vi "Kamera hinten.vi"() -> (0 "Paket erkannt":bool, 1 "Barcode erkannt":bool, 2 "Paketkoordinaten":cluster{"X":dbl, "Y":dbl}, 3 "Barcode":u32)   [LabVIEW 2019]
doc: "Erkennt mit Hilfe der hiten angebrachten Kamera das Paket und den Barcode. Es gitb den Barcode aus und eine ungefähre mittige Position der Kamera."
panel:
  out "Rectangles (Shape Detection 1)":T1(array[cluster]) {"Corners"."Y" format="%.2f"; "Corners"."X" format="%.2f"}
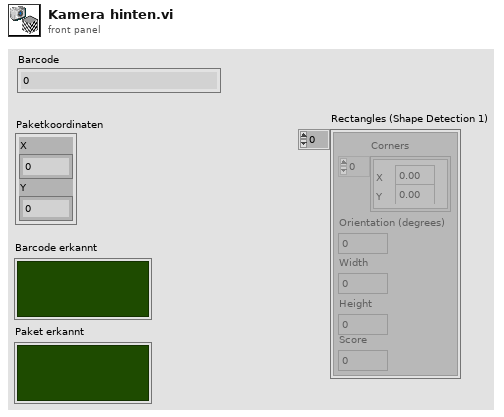
[diagram p1: front panel]
types:
  T1 = cluster{"Corners":cluster{"X":sgl, "Y":sgl}[], "Orientation (degrees)":dbl, "Width":dbl, "Height":dbl, "Score":dbl}[]
  T2 = typedef "IMAQ Image.ctl" = refnum<image>
  T3 = typedef "Edge New.ctl" = cluster{"Location (Pixel)":cluster{"X":sgl, "Y":sgl}, "Location (Real-World)":cluster{"X":sgl, "Y":sgl}, "Distance (Pixel)":dbl, "Distance (Real-World)":dbl, "Strength":dbl, "Noise":dbl, "Rising?":bool}
  T4 = cluster{"Data":string, "Special Char 1":string, "Special Char 2":string, "Checksum(s)":string, "Barcode Type":u32, "Confidence Level":sgl, "Bounding Box":cluster{"x":sgl, "y":sgl}[]}[]
  T5 = cluster{"Edge Information (Edge Detector 3)[0]":T3, "Edge Information (Edge Detector 3)[1]":T3, "Edge Information (Edge Detector 3)[2]":T3, "Edge Information (Edge Detector 3)[3]":T3, "Edge Information (Edge Detector 3)[4]":T3, "Edge Information (Edge Detector 3)[5]":T3, "Edge Information (Edge Detector 3)[6]":T3, "Edge Information (Edge Detector 3)[7]":T3, "Edge Information (Edge Detector 3)[8]":T3}
  T6 = cluster{"Barcodes (Barcode Reader 1)[0]":cluster{"Data":string, "Special Char 1":string, "Special Char 2":string, "Checksum(s)":string, "Barcode Type":u32, "Confidence Level":sgl, "Bounding Box":cluster{"x":sgl, "y":sgl}[]}, "Barcodes (Barcode Reader 1)[1]":cluster{"Data":string, "Special Char 1":string, "Special Char 2":string, "Checksum(s)":string, "Barcode Type":u32, "Confidence Level":sgl, "Bounding Box":cluster{"x":sgl, "y":sgl}[]}, "Barcodes (Barcode Reader 1)[2]":cluster{"Data":string, "Special Char 1":string, "Special Char 2":string, "Checksum(s)":string, "Barcode Type":u32, "Confidence Level":sgl, "Bounding Box":cluster{"x":sgl, "y":sgl}[]}, "Barcodes (Barcode Reader 1)[3]":cluster{"Data":string, "Special Char 1":string, "Special Char 2":string, "Checksum(s)":string, "Barcode Type":u32, "Confidence Level":sgl, "Bounding Box":cluster{"x":sgl, "y":sgl}[]}, "Barcodes (Barcode Reader 1)[4]":cluster{"Data":string, "Special Char 1":string, "Special Char 2":string, "Checksum(s)":string, "Barcode Type":u32, "Confidence Level":sgl, "Bounding Box":cluster{"x":sgl, "y":sgl}[]}, "Barcodes (Barcode Reader 1)[5]":cluster{"Data":string, "Special Char 1":string, "Special Char 2":string, "Checksum(s)":string, "Barcode Type":u32, "Confidence Level":sgl, "Bounding Box":cluster{"x":sgl, "y":sgl}[]}, "Barcodes (Barcode Reader 1)[6]":cluster{"Data":string, "Special Char 1":string, "Special Char 2":string, "Checksum(s)":string, "Barcode Type":u32, "Confidence Level":sgl, "Bounding Box":cluster{"x":sgl, "y":sgl}[]}, "Barcodes (Barcode Reader 1)[7]":cluster{"Data":string, "Special Char 1":string, "Special Char 2":string, "Checksum(s)":string, "Barcode Type":u32, "Confidence Level":sgl, "Bounding Box":cluster{"x":sgl, "y":sgl}[]}, "Barcodes (Barcode Reader 1)[8]":cluster{"Data":string, "Special Char 1":string, "Special Char 2":string, "Checksum(s)":string, "Barcode Type":u32, "Confidence Level":sgl, "Bounding Box":cluster{"x":sgl, "y":sgl}[]}}
  T7 = cluster{"Edge Information (Edge Detector 2)[0]":T3, "Edge Information (Edge Detector 2)[1]":T3, "Edge Information (Edge Detector 2)[2]":T3, "Edge Information (Edge Detector 2)[3]":T3, "Edge Information (Edge Detector 2)[4]":T3, "Edge Information (Edge Detector 2)[5]":T3, "Edge Information (Edge Detector 2)[6]":T3, "Edge Information (Edge Detector 2)[7]":T3, "Edge Information (Edge Detector 2)[8]":T3}
  T8 = cluster{"Data":string, "Special Char 1":string, "Special Char 2":string, "Checksum(s)":string, "Barcode Type":u32, "Confidence Level":sgl, "Bounding Box":cluster{"x":sgl, "y":sgl}[]}
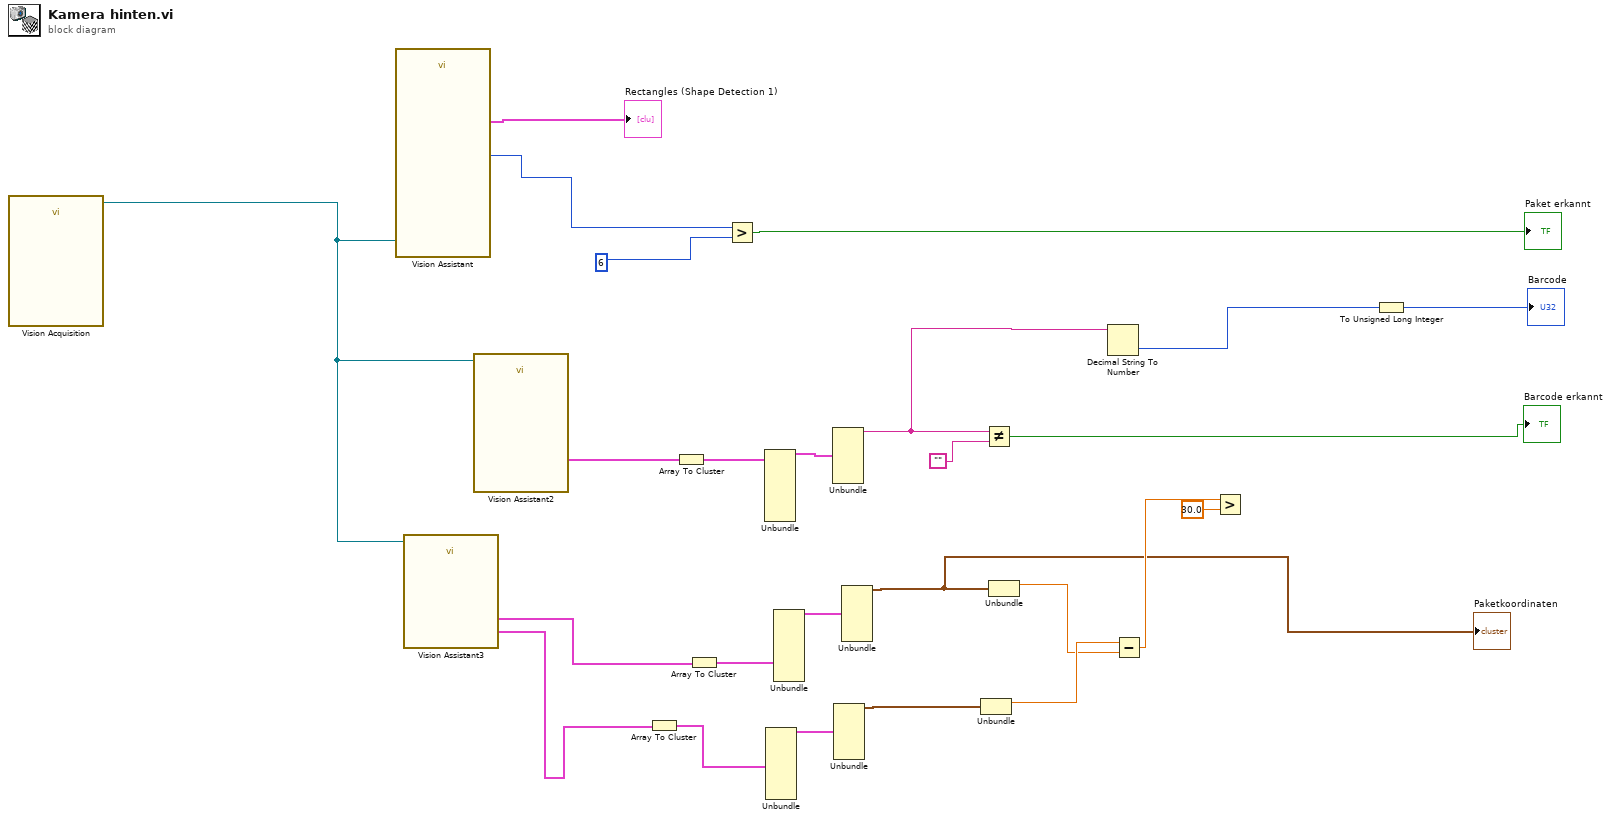
[diagram p0: block diagram]
diagram:
  n1 = call "Vision Acquisition"() -> ("Image Out"=w14:T2)  [unwired: 24 in, 3 out]
  n2 = call "Vision Assistant"("Image In"=w14) -> ("Rectangles (Shape Detection 1)"=→"Rectangles (Shape Detection 1)":T1, "Number of Matches (Shape Detection 1)"=w8:i32)  [unwired: 22 in, 3 out]
  n3 = call "Vision Assistant3"("Image In"=w14) -> ("Edge Information (Edge Detector 2)"=w17:T3[], "Edge Information (Edge Detector 3)"=w21:T3[])  [unwired: 23 in, 2 out]
  n4 = call "Vision Assistant2"("Image In"=w14) -> ("Barcodes (Barcode Reader 1)"=w10:T4)  [unwired: 22 in, 4 out]
  n5 = Array To Cluster(array=w21) -> (cluster=w20:T5)
  n6 = Array To Cluster(array=w10) -> (cluster=w11:T6)
  n7 = Array To Cluster(array=w17) -> (cluster=w15:T7)
  n8 = Greater?(x=w8, y=6) -> (0:→"Paket erkannt":bool)
  n9 = Unbundle(w11) -> ("Barcodes (Barcode Reader 1)[0]"=w12:T8)  [unwired: 8 out]
  n10 = Unbundle(w20) -> ("Edge Information (Edge Detector 3)[0]"=w19:T3)  [unwired: 8 out]
  n11 = Unbundle(w15) -> ("Edge Information (Edge Detector 2)[0]"=w16:T3)  [unwired: 8 out]
  n12 = Unbundle(w12) -> ("Data"=w3:string)  [unwired: 6 out]
  n13 = Unbundle(w19) -> ("Location (Pixel)"=w18:cluster{"X":sgl, "Y":sgl})  [unwired: 6 out]
  n14 = Unbundle(w16) -> ("Location (Pixel)"=w4:cluster{"X":sgl, "Y":sgl})  [unwired: 6 out]
  "Paketkoordinaten" <- w4
  n15 = Unbundle(w18) -> ("X"=w23:sgl)  [unwired: 1 out]
  n16 = Not Equal?(x=w3, y="") -> (x != y?=→"Barcode erkannt":bool)
  n17 = Unbundle(w4) -> ("X"=w22:sgl)  [unwired: 1 out]
  n18 = Decimal String To Number(string=w3) -> (number=w2:i32)  [unwired: 2 in, 1 out]
  n19 = Subtract(x=w23, y=w22) -> (x-y=w25:sgl)
  n20 = Greater?(x=w25, y=30.0) -> ()  [unwired: 1 out]
  n21 = To Unsigned Long Integer(number=w2) -> (unsigned 32bit integer=→"Barcode":u32)
